vi "Load Calibration Flow Settings Tables.vi"() -> (0 "stage 4 - span":i16[][](array[numeric])=[[0, 3, 500, 1, 1], [1, 3, 500, 1, 1], [2, 3, 500, 1, 1], [3, 3, 500, 1, 1], [4, 3, 500, 1, 1], [5, 3, 500, 1, 1], [6, 3, 500, 1, 1], [7, 3, 500, 0, 0], [8, 3, 500, 0, 0], [9, 3, 500, 0, 0], [10, 3, 500, 0, 0], [11, 3, 500, 0, 0], [12, 3, 500, 0, 0], [13, 3, 500, 0, 0], [14, 3, 500, 0, 0], [15, 3, 500, 0, 0], [16, 3, 500, 0, 0], [17, 3, 500, 0, 0], [18, 3, 500, 0, 0], [19, 3, 500, 0, 0], [20, 3, 500, 0, 0], [21, 3, 500, 0, 0], [22, 3, 500, 0, 0], [23, 3, 500, 0, 0], [24, 3, 500, 0, 0], [25, 3, 500, 0, 0], [26, 3, 500, 0, 0], [27, 3, 500, 0, 0], [28, 3, 500, 0, 0], [29, 3, 500, 0, 0], [30, 3, 500, 0, 0], [31, 3, 500, 0, 0], [32, 3, 500, 0, 0], [33, 3, 500, 0, 0], [34, 3, 500, 0, 0], [35, 3, 500, 0, 0], [36, 3, 500, 0, 0], [37, 3, 500, 0, 0], [38, 3, 500, 0, 0], [39, 3, 500, 0, 0], [40, 3, 500, 0, 0], [41, 3, 500, 0, 0], [42, 3, 500, 0, 0], [43, 3, 500, 0, 0], [44, 3, 500, 0, 0], [45, 3, 500, 0, 0], [46, 3, 500, 0, 0], [47, 3, 500, 0, 0], [48, 3, 500, 0, 0], [49, 3, 500, 0, 0], [50, 3, 500, 0, 0], [51, 3, 500, 0, 0], [52, 3, 500, 0, 0], [53, 3, 500, 0, 0], [54, 3, 500, 0, 0], [55, 3, 500, 0, 0], [56, 3, 500, 0, 0], [57, 3, 500, 0, 0], [58, 3, 500, 0, 0], [59, 3, 500, 0, 0], [60, 3, 500, 0, 0], [61, 3, 500, 0, 0], [62, 3, 500, 0, 0], [63, 3, 500, 0, 0], [64, 3, 500, 0, 0], [65, 3, 500, 0, 0], [66, 3, 500, 0, 0], [67, 3, 500, 0, 0], [68, 3, 500, 0, 0], [69, 3, 500, 0, 0], [70, 3, 500, 0, 0], [71, 3, 500, 0, 0], [72, 3, 500, 0, 0], [73, 3, 500, 0, 0], [74, 3, 500, 0, 0], [75, 3, 500, 0, 0], [76, 3, 500, 0, 0], [77, 3, 500, 0, 0], [78, 3, 500, 0, 0], [79, 3, 500, 0, 0], [80, 3, 500, 0, 0], [81, 3, 500, 0, 0], [82, 3, 500, 0, 0], [83, 3, 500, 0, 0], [84, 3, 500, 0, 0], [85, 3, 500, 0, 0], [86, 3, 500, 0, 0], [87, 3, 500, 0, 0], [88, 3, 500, 0, 0], [89, 3, 500, 0, 0], [90, 3, 500, 0, 0], [91, 3, 500, 0, 0], [92, 3, 50, 1, 1]], 1 "stage 3 - high":i16[][](array[numeric])=[[0, 3, 500, 0, 1], [1, 3, 500, 0, 1], [2, 3, 500, 0, 1], [3, 3, 500, 0, 1], [4, 3, 500, 0, 1], [5, 3, 500, 0, 1], [6, 3, 50, 0, 1]], 2 "stage 2 - zeroing":i16[][](array[numeric])=[[0, 2, 500, 1, 0], [1, 2, 500, 1, 0], [2, 2, 500, 1, 0], [3, 2, 500, 1, 0], [4, 2, 500, 1, 0], [5, 2, 500, 1, 0], [6, 2, 50, 1, 0]], 3 "stage1 - humidity check":i16[][](array[numeric])=[[0, 1, 500, 1, 0], [1, 1, 50, 1, 0], [2, 1, 50, 1, 0], [3, 1, 50, 1, 0], [4, 1, 50, 1, 0], [5, 1, 50, 1, 0], [6, 1, 100, 0, 1], [7, 1, 150, 0, 1], [8, 1, 200, 0, 1], [9, 1, 250, 1, 0], [10, 1, 300, 1, 1], [0, 1, 350, 0, 0]], 4 "stage 5 - offset adjust":i16[][](array[numeric]), 5 "termination array - should be just one row of zeros":i16[][](array[numeric]))   [LabVIEW 2016]
panel:
  out "Indeces":u16[](array[numeric])
  out "text array":string[][](array[string])
  out "all rows":sgl[][](array[numeric])
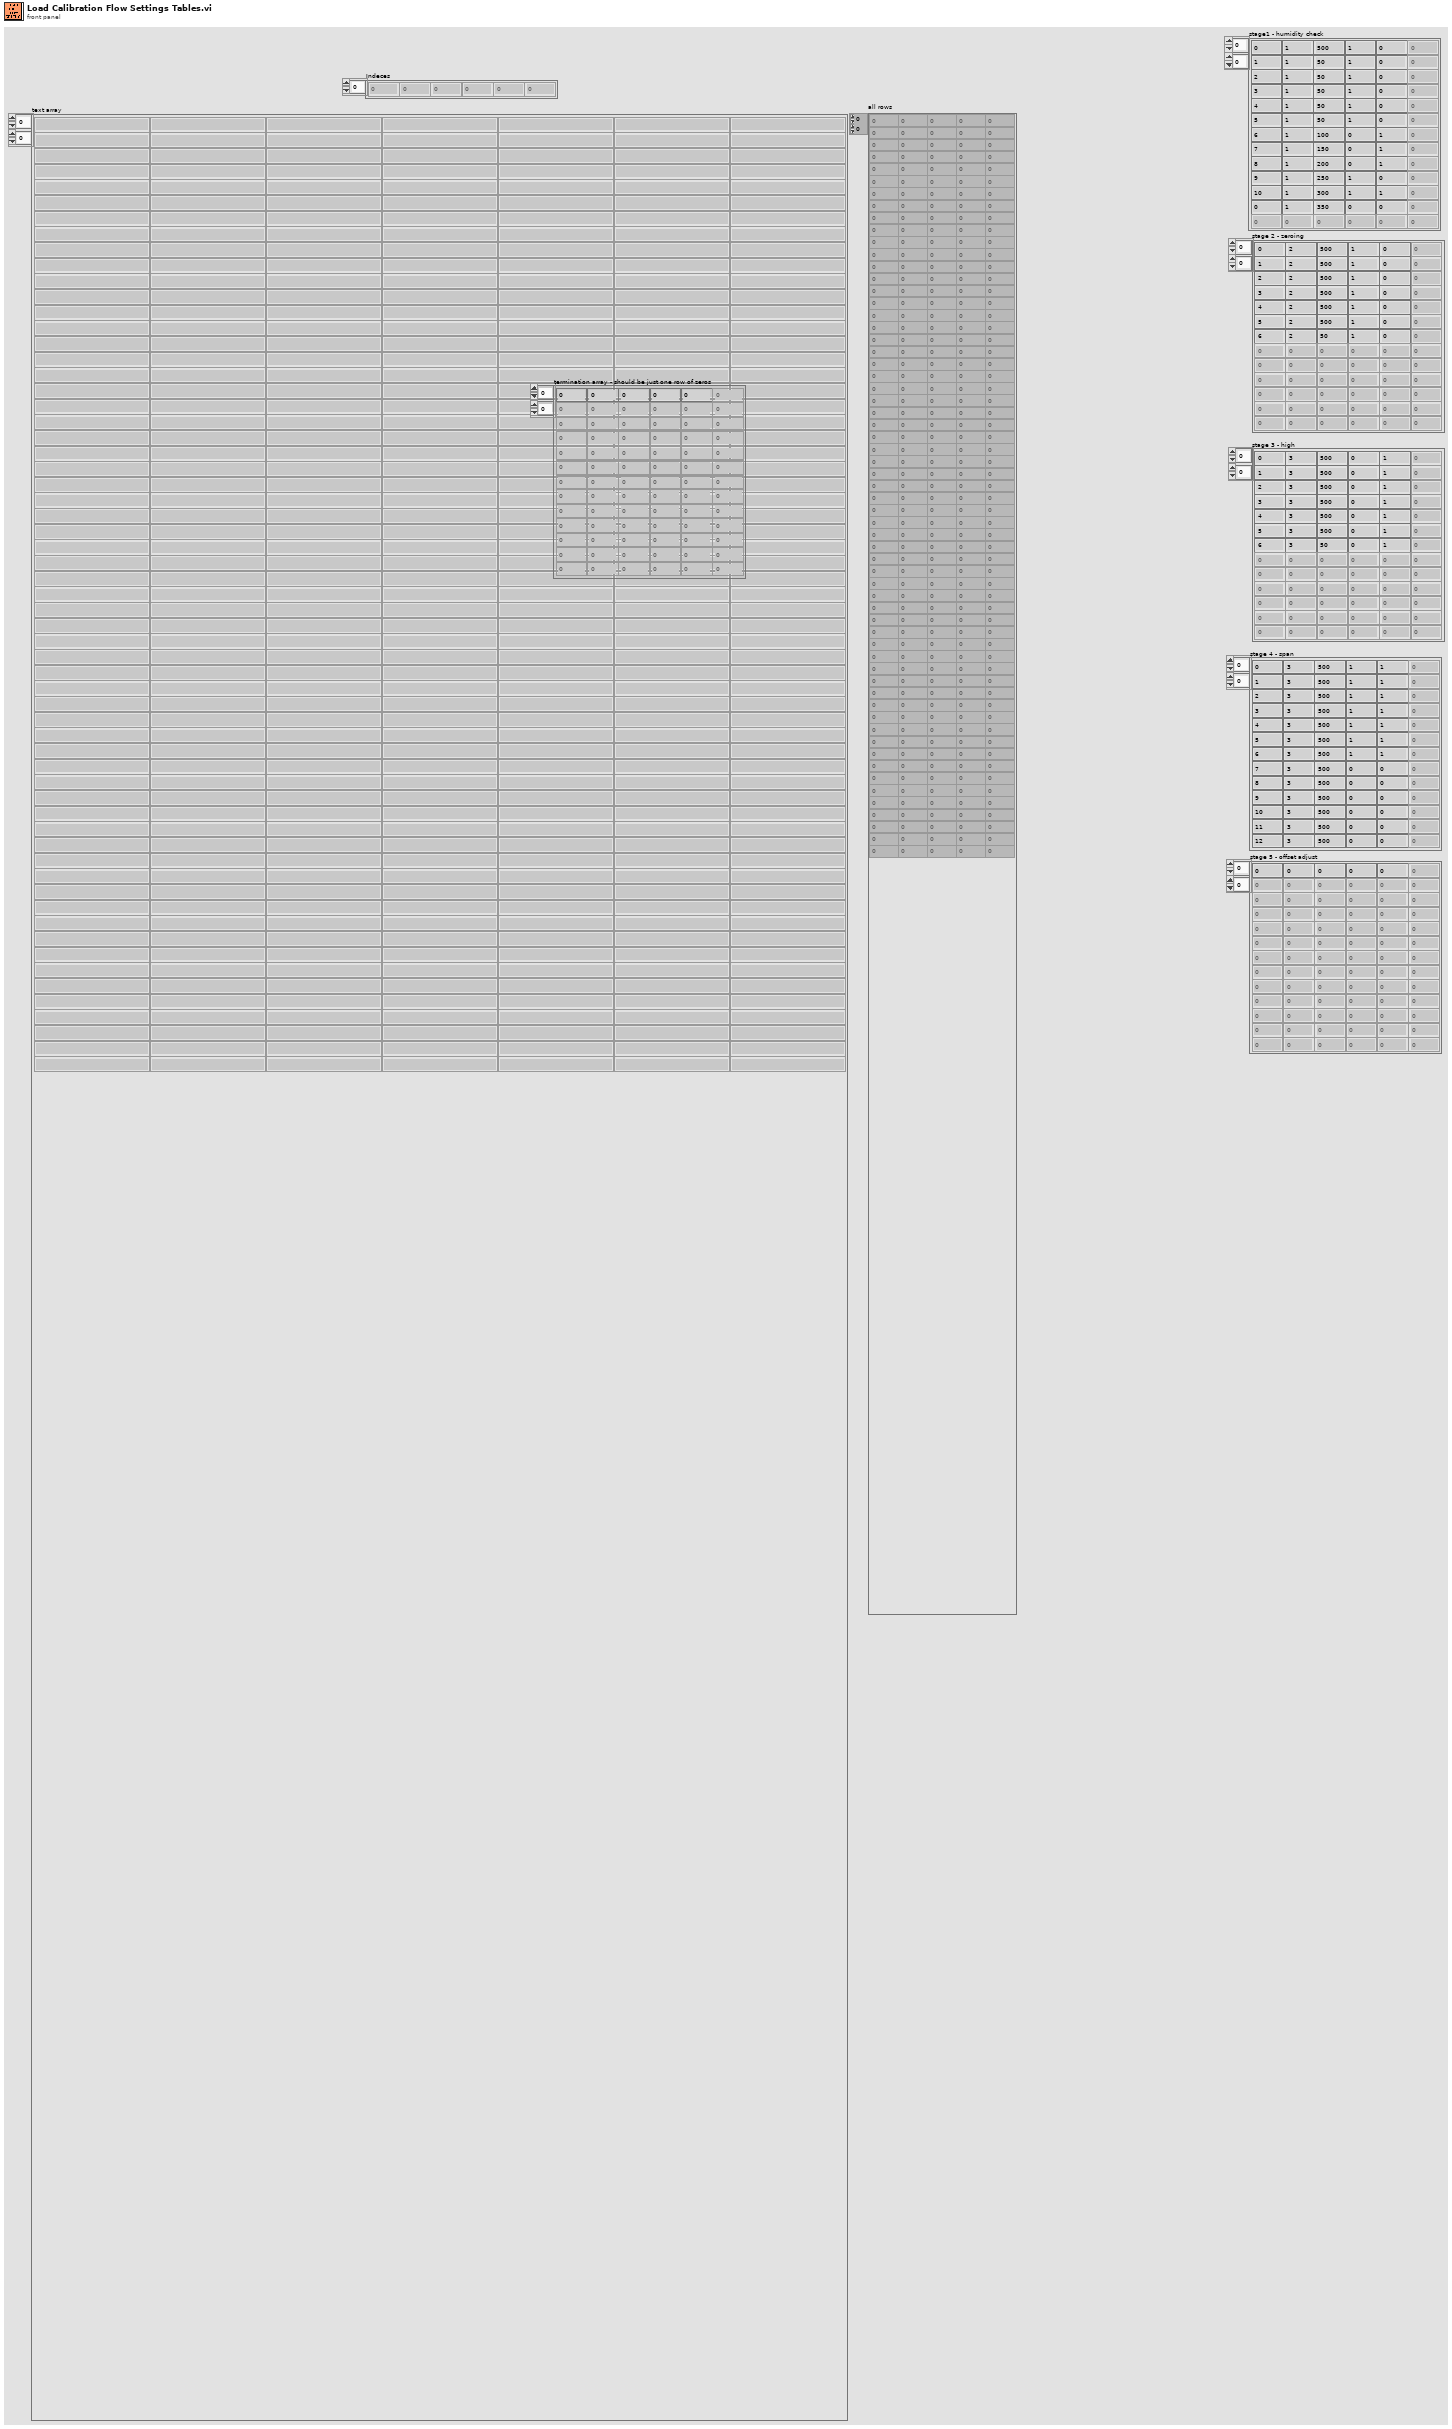
[diagram p1: front panel]
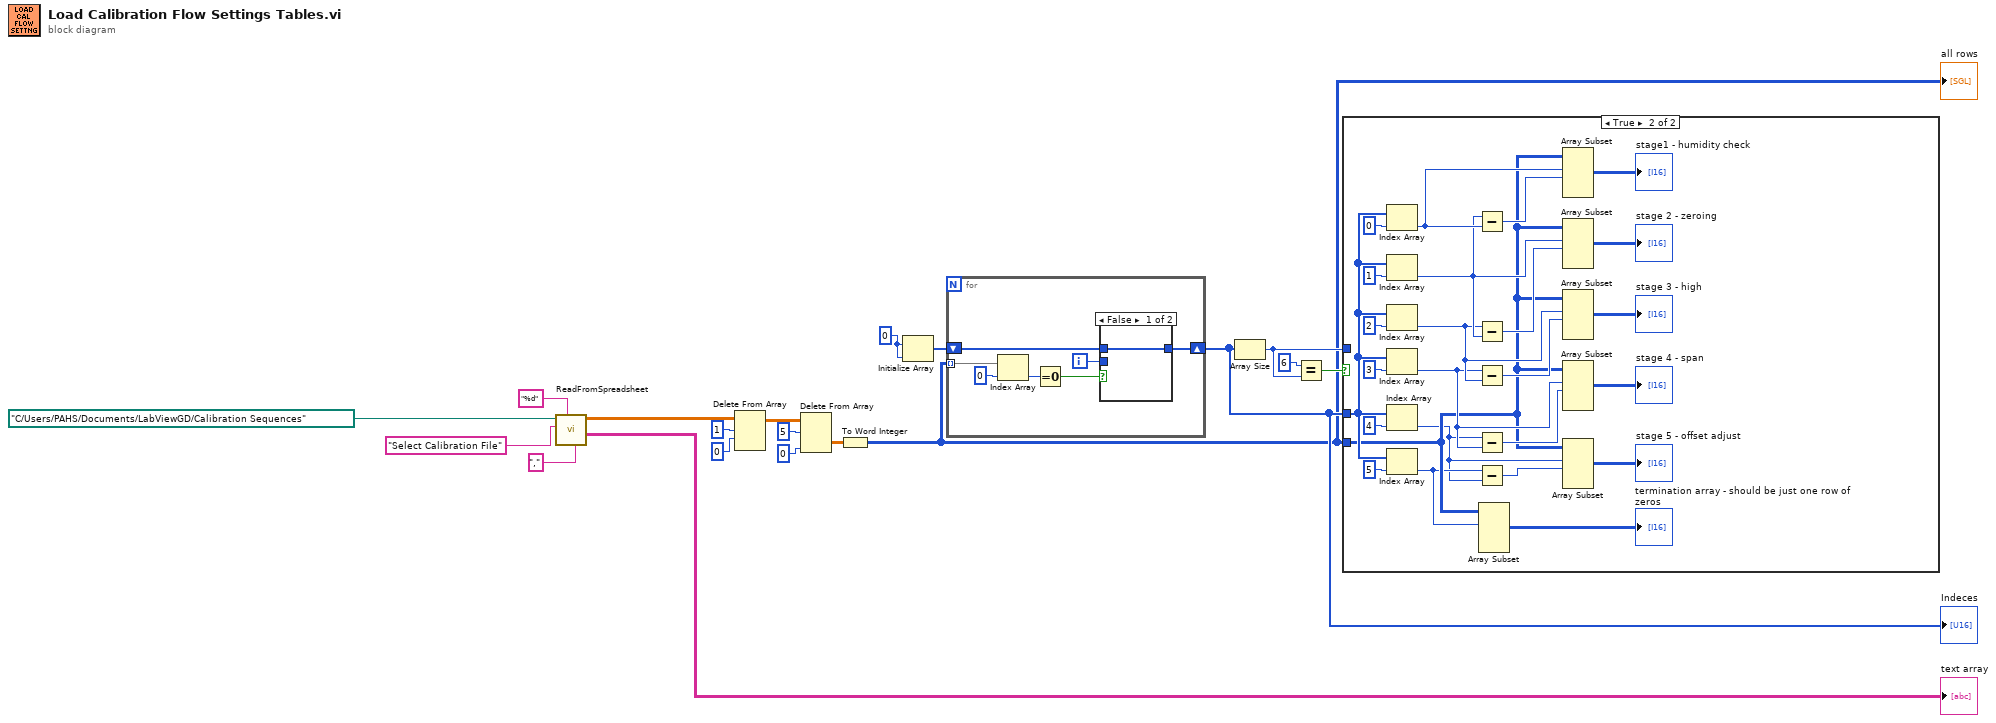
[diagram p0: block diagram]
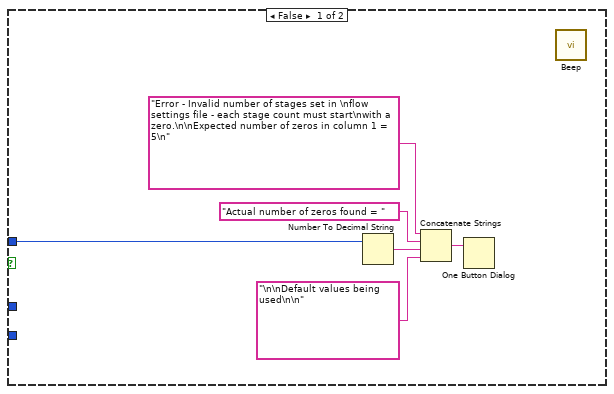
[diagram p2: hidden frame]
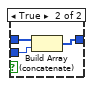
[diagram p3: hidden frame]
diagram:
  w9 = 0
  n1 = call "ReadFromSpreadsheet.vi"("delimiter (\\t)"="," ("delimiter (\\t)"), "format (%d)"="%d", "File Prompt"="Select Calibration File", "file path"=path "C:/Users/PAHS/Documents/LabViewGD/Calibration Sequences") -> ("text array"=→"text array":string[][], "all rows"=w16:sgl[][])  [unwired: 3 in, 3 out]
  n2 = Delete From Array(array=w16, length=1, index (row)=0) -> (array with subset deleted=w12:sgl[][])  [unwired: 1 in, 1 out]
  n3 = Delete From Array(array=w12, length=5, index (col)=0 ("index (row)")) -> (deleted portion=w5:sgl[][])  [unwired: 1 in, 1 out]
  n4 = To Word Integer(number=w5) -> (16bit integer=w3:i16[][])
  "all rows" <- w3
  n5 = Initialize Array(w9, w9) -> (w10:i32[])
  n6 = for {
    tunnel: w3 -> [w25] mode=indexing
    shift-right: [w20] -> w4
    shift-left: w10 -> [w21]
    i -> [w22]
    n7 = Index Array(array=w25, index=0) -> (element=w24:i16)
    n8 = Equal To 0?(x=w24) -> (x = 0?=w23:bool)
    n9 = case shown="False" w23 {
      tunnel: w22 -> [_ w29]
      tunnel: w21 -> [w27 w30]
      tunnel: [w27 w28] -> w20
      frame False {
      }
      frame True {
        n10 = Build Array (concatenate)(w30, w29) -> (w28:i32[])
      }
    }
  }
  "Indeces" <- w4
  n11 = Array Size(array=w4) -> (size(s)=w6:i32)
  n12 = Equal?(x=6, y=w6) -> (x = y?=w7:bool)
  n13 = case shown="True" w7 {
    tunnel: w6 -> [w32 _]
    tunnel: w3 -> [_ w40]
    tunnel: w4 -> [_ w42]
    frame False {
      n14 = Number To Decimal String(number=w32) -> (decimal integer string=w31:string)  [unwired: 1 in]
      n15 = Concatenate Strings("Error - Invalid number of stages set in \nflow settings file - each stage count must start\nwith a zero.\n\nExpected number of zeros in column 1 = 5\n" ("message"), "Actual number of zeros found = " ("string"), w31, "\n\nDefault values being used\n\n" ("string")) -> (w33:string)
      n16 = One Button Dialog(message=w33) -> ()  [unwired: 1 in, 1 out]
      n17 = call <vilib>:"Beep.vi"() -> ()  [unwired: 12 in]
    }
    frame True {
      n18 = Index Array(array=w42, index=0) -> (element=w47:i32)
      n19 = Index Array(array=w42, index=1) -> (element=w46:i32)
      n20 = Index Array(array=w42, index=2) -> (element=w45:i32)
      n21 = Index Array(array=w42, index=3) -> (element=w44:i32)
      n22 = Index Array(array=w42, index=4) -> (element=w38:i32)
      n23 = Index Array(array=w42, index=5) -> (element=w39:i32)
      n24 = Subtract(x=w46, y=w47) -> (x-y=w52:i32)
      n25 = Subtract(x=w45, y=w46) -> (x-y=w49:i32)
      n26 = Subtract(x=w44, y=w45) -> (x-y=w50:i32)
      n27 = Subtract(x=w38, y=w44) -> (x-y=w51:i32)
      n28 = Subtract(x=w39, y=w38) -> (x-y=w37:i32)
      n29 = Array Subset(array=w40, index (row)=w39) -> (→"termination array - should be just one row of zeros":i16[][])  [unwired: 3 in]
      n30 = Array Subset(array=w40, index (row)=w47, length (row)=w52) -> (→"stage1 - humidity check":i16[][])  [unwired: 2 in]
      n31 = Array Subset(array=w40, index (row)=w46, length (row)=w49) -> (→"stage 2 - zeroing":i16[][])  [unwired: 2 in]
      n32 = Array Subset(array=w40, index (row)=w45, length (row)=w50) -> (→"stage 3 - high":i16[][])  [unwired: 2 in]
      n33 = Array Subset(array=w40, index (row)=w44, length (row)=w51) -> (→"stage 4 - span":i16[][])  [unwired: 2 in]
      n34 = Array Subset(array=w40, index (row)=w38, length (row)=w37) -> (→"stage 5 - offset adjust":i16[][])  [unwired: 2 in]
    }
  }
